vi "h.ACQ.SetEnableSpectrumStreaming.vi"(8 "error in":errorcluster, 9 "Timeout (ms)":i32=10000, 10 "Enable":bool, 11 "Connection ID in":refnum<k5>) -> (0 "error out":errorcluster, 3 "Connection ID out":refnum<k5>)   [LabVIEW 2016, in "h.Library.lvlib"]
uses:
  h.Library.lvlib
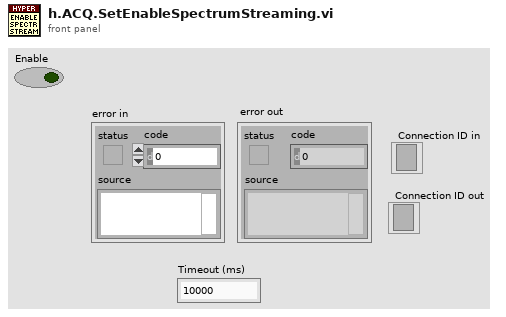
[diagram p1: front panel]
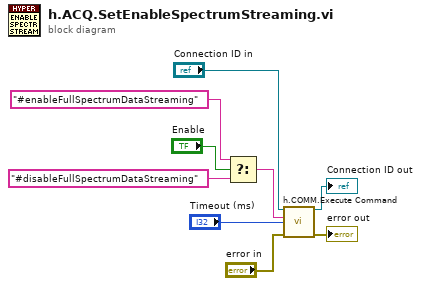
[diagram p0: block diagram]
diagram:
  n1 = Select(t="#enableFullSpectrumDataStreaming" ("Command"), s="Enable", f="#disableFullSpectrumDataStreaming" ("Command")) -> (s? t:f=w6:string)
  n2 = call "h.COMM.Execute Command.vi"("Connection ID"="Connection ID in", "Command"=w6, "Timeout"="Timeout (ms)", "error in"="error in") -> ("Connection ID out"=→"Connection ID out":refnum<k5>, "error out"=→"error out":errorcluster)  [unwired: 4 in, 6 out]
